vi "Run.vi"(0 "object in":refnum<class "Logger.lvclass">, 5 "error in (no error)":errorcluster) -> (14 "object out":refnum<class "Logger.lvclass">, 19 "error out":errorcluster)   [LabVIEW 2014, in "Logger.lvclass"]
uses:
  Logger.lvclass
  Logger.lvclass/Logger.ctl
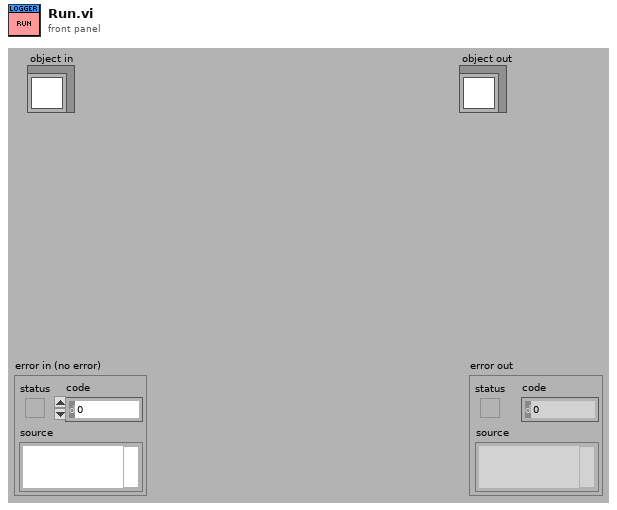
[diagram p1: front panel]
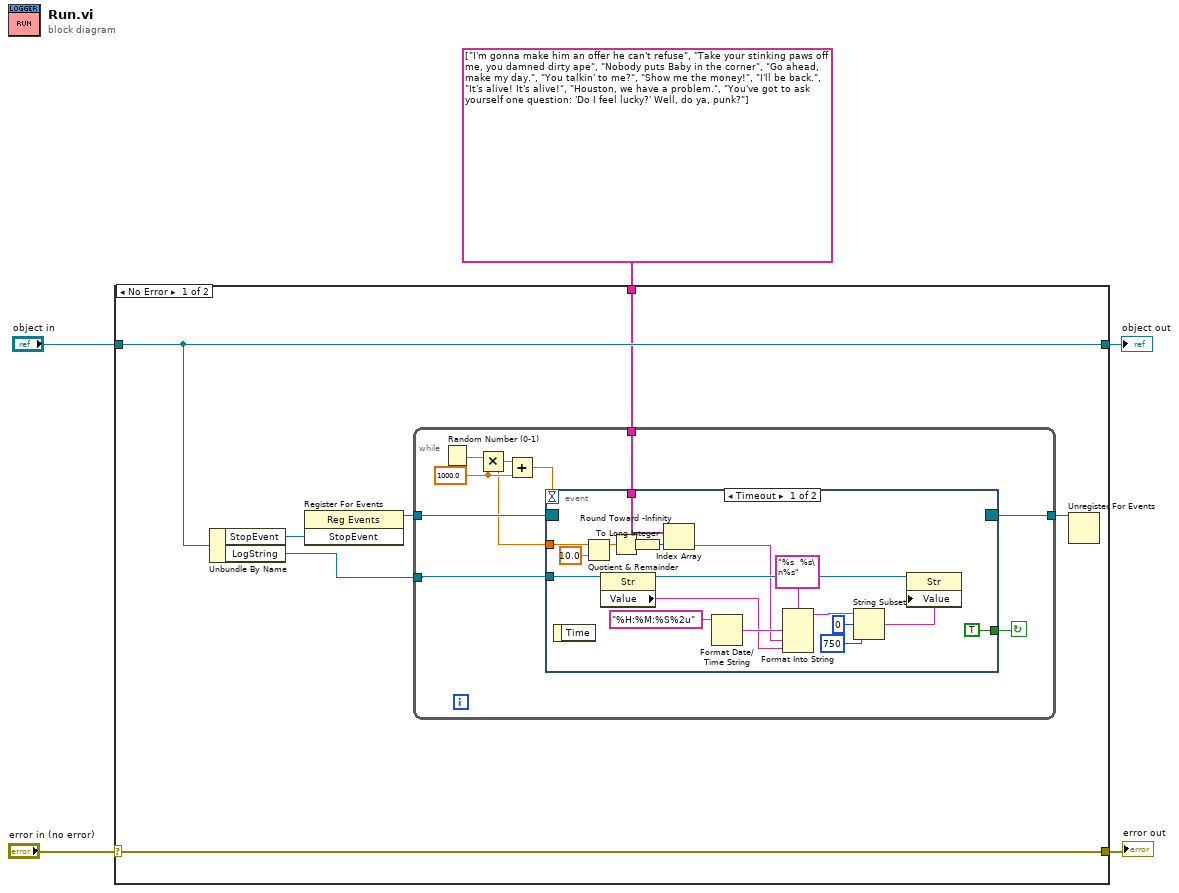
[diagram p0: block diagram]
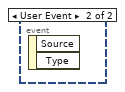
[diagram p2: hidden frame]
diagram:
  n1 = case shown="No Error" "error in (no error)" {
    selector: "error in (no error)" -> [w12 w41]
    tunnel: [w12 w41] -> w4
    tunnel: [w8 w40] -> w2
    tunnel: "object in" -> [w8 w40]
    tunnel: string[] ["I'm gonna make him an offer he can't refuse", "Take your stinking paws off me, you damned dirty ape", "Nobody puts Baby in the corner", "Go ahead, make my day.", "You talkin' to me?", "Show me the money!", "I'll be back.", "It's alive! It's alive!", "Houston, we have a problem.", "You've got to ask yourself one question: 'Do I feel lucky?' Well, do ya, punk?"] -> [w7 _]
    frame No Error {
      n2 = Unbundle By Name(w8) -> ("StopEvent"=w10:refnum<user-event>, "LogString"=w9:refnum<vi>)
      n3 = register-events(w10) -> (reference out=w11:refnum<event-registration>)  [unwired: 2 in, 1 out]
      n4 = while {
        tunnel: w11 -> [w21]
        tunnel: w9 -> [w15]
        tunnel: w7 -> [w14]
        tunnel: [w13] -> w6
        stop <- w20 continue-if-true
        w19 = 1000.0 ("y")
        n5 = Random Number (0-1)() -> (number: 0 to 1=w17:dbl)
        n6 = Multiply(x=w17, y=w19) -> (x*y=w16:dbl)
        n7 = Add(x=w16, y=w19) -> (x+y=w18:dbl)
        n8 = event shown="[0] Timeout" {
          selector: w21 -> [_ _]
          dyn-events: [_ _] -> w13
          timeout: w18 -> [_ _]
          tunnel: [TRUE _] -> w20
          tunnel: w16 -> [w24 _]
          tunnel: w15 -> [w36 _]
          tunnel: w14 -> [w31 _]
          event Timeout {
            n9 = event-data() -> ()  [unwired: 1 in, 1 out]
            n10 = Quotient & Remainder(x=w24, y=10.0) -> (x-y*floor(x/y)=w25:dbl)  [unwired: 1 out]
            n11 = property class="Str"(reference=w36) -> (reference out=w38:refnum<vi>, "Value"=w32:string)  [unwired: 1 in, 1 out]
            n12 = Round Toward -Infinity(1:w25) -> (0:w23:dbl)
            n13 = To Long Integer(number=w23) -> (32bit integer=w22:i32)
            n14 = Index Array(array=w31, index=w22) -> (element=w30:string)
            n15 = Format Date/Time String(time format string (%c)="%H:%M:%S%2u") -> (date/time string=w34:string)  [unwired: 2 in]
            n16 = Format Into String(format string="%s  %s\n%s", w34, w30, w32) -> (resulting string=w27:string)  [unwired: 2 in, 1 out]
            n17 = String Subset(string=w27, offset (0)=0, length (rest)=750 ("length (rest)")) -> (substring=w26:string)
            n18 = property class="Str"(reference=w38, "Value"=w26) -> ()  [unwired: 1 in, 2 out]
          }
          event User Event {
            n19 = event-data() -> ()  [unwired: 1 in, 2 out]
          }
        }
      }
      n20 = Unregister For Events(event registration refnum=w6) -> ()  [unwired: 1 in, 1 out]
    }
    frame Error {
    }
  }
  "error out" <- w4
  "object out" <- w2
